vi "calculator.vi"() -> ()   [LabVIEW 2015]
panel:
  out "time to use(s)":dbl
  in  "1":bool
  in  "stop":bool
  in  "CE":bool
  in  "backspace":bool
  in  "1/x":bool
  in  "+/-":bool
  in  "sqrt":bool
  in  ".":bool
  out "message":string
  out "show":string
  in  "C":bool
  out "Current Time":timestamp
  in  "=":bool
  in  "/":bool
  in  "*":bool
  in  "-":bool
  in  "+":bool
  in  "0":bool
  in  "9":bool
  in  "8":bool
  in  "7":bool
  in  "6":bool
  in  "5":bool
  in  "4":bool
  in  "3":bool
  in  "2":bool
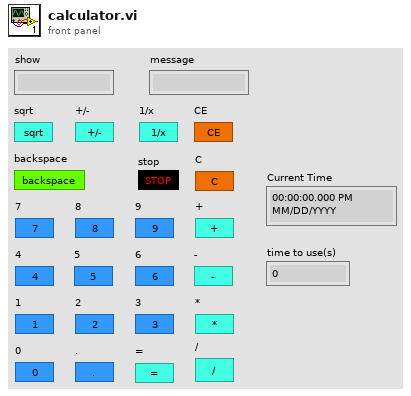
[diagram p1: front panel]
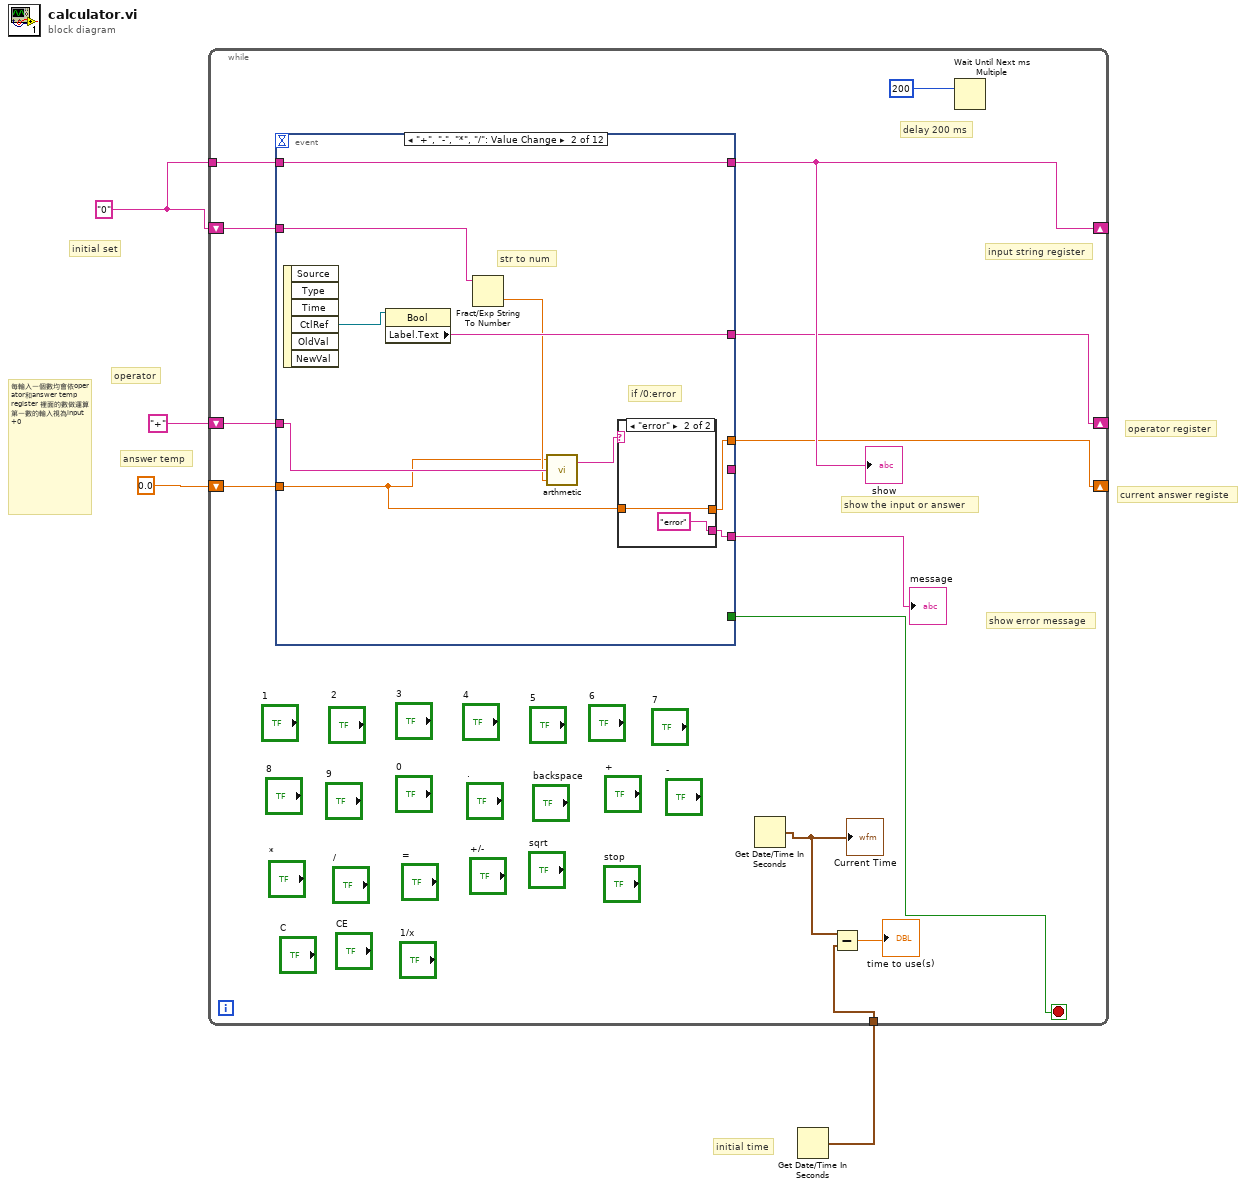
[diagram p0: block diagram]
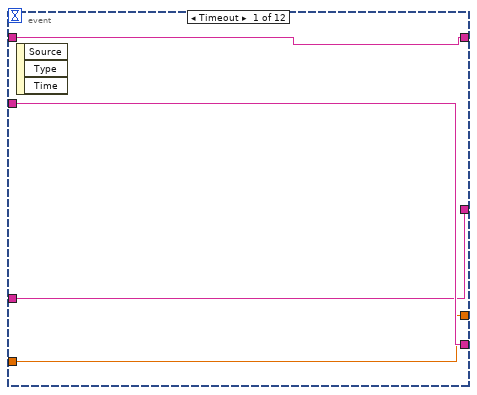
[diagram p2: hidden frame]
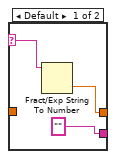
[diagram p3: hidden frame]
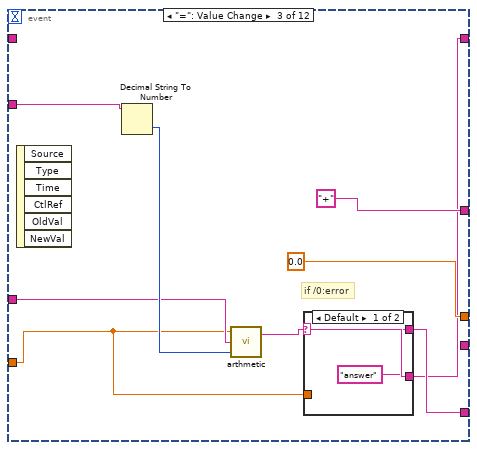
[diagram p4: hidden frame]
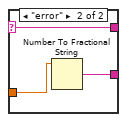
[diagram p5: hidden frame]
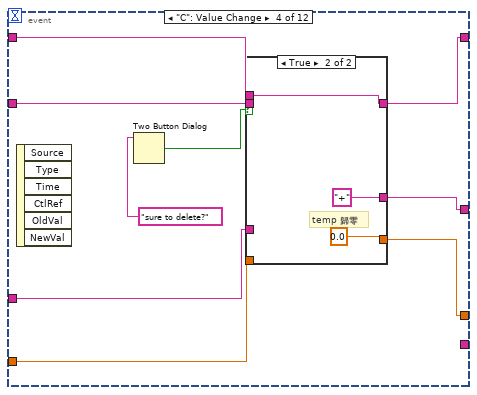
[diagram p6: hidden frame]
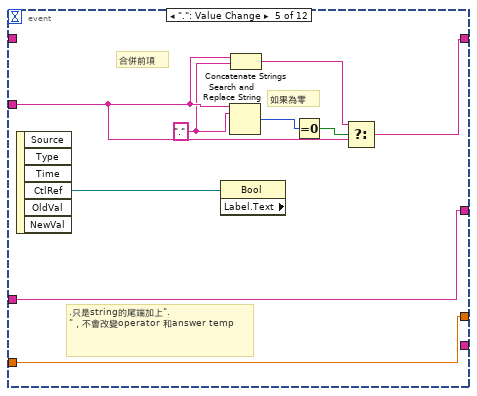
[diagram p8: hidden frame]
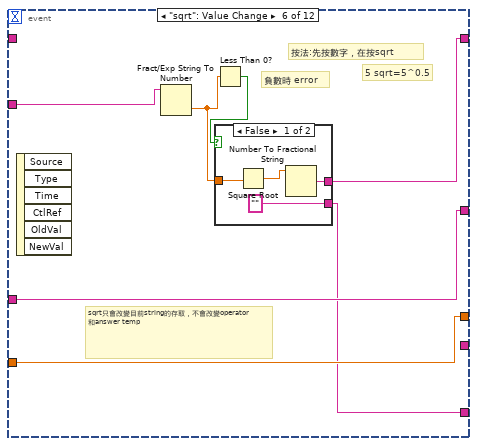
[diagram p9: hidden frame]
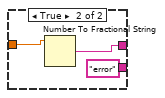
[diagram p10: hidden frame]
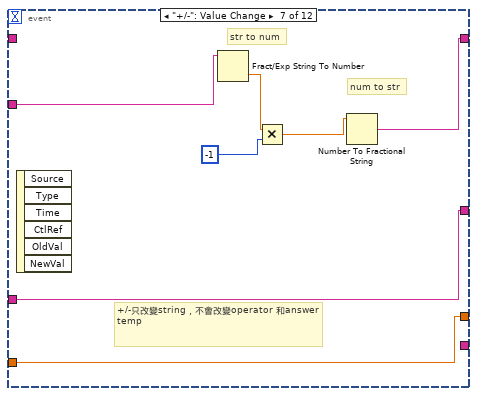
[diagram p11: hidden frame]
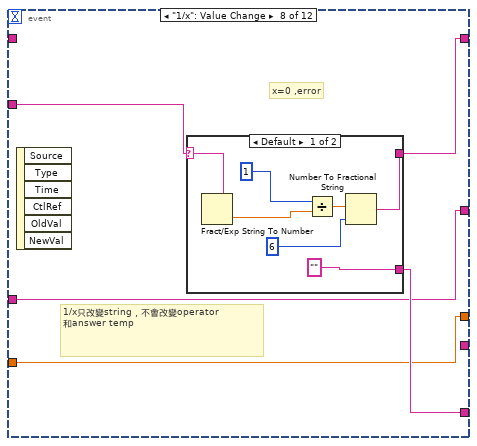
[diagram p12: hidden frame]
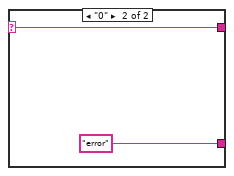
[diagram p13: hidden frame]
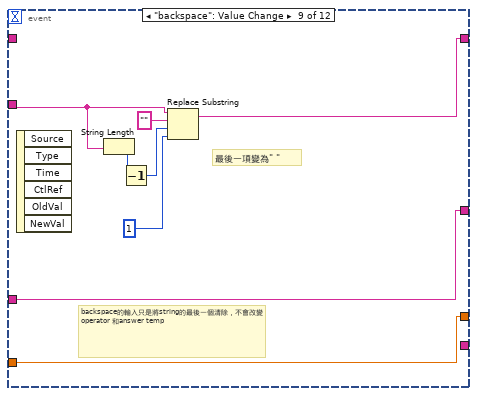
[diagram p14: hidden frame]
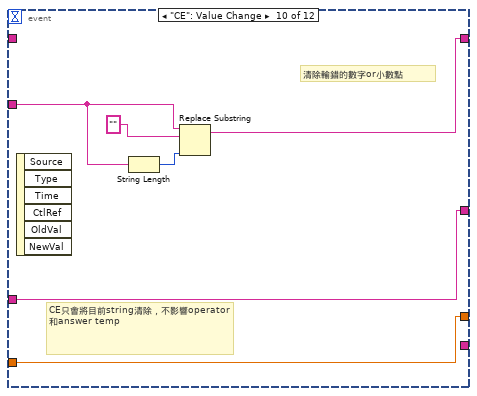
[diagram p15: hidden frame]
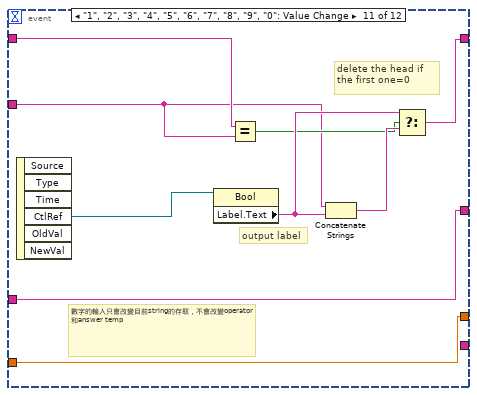
[diagram p16: hidden frame]
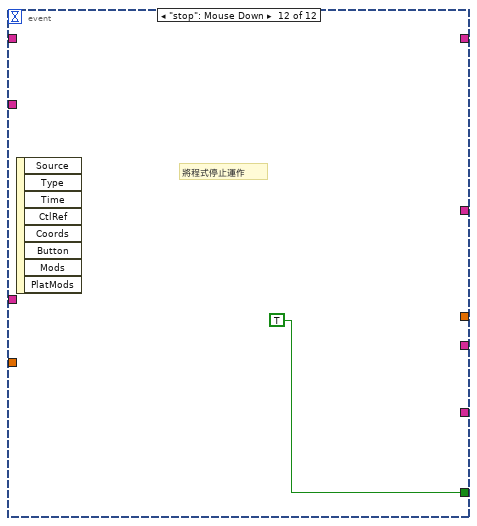
[diagram p17: hidden frame]
diagram:
  w3 = "0"
  # "每輸入一個數均會依operator和answer temp register 裡面的數做運算\n第一數的輸入視為input+0"
  # "current answer registe"
  # "operator register"
  # "answer temp"
  # "operator"
  # "initial time"
  # "initial set"
  n1 = Get Date/Time In Seconds() -> (seconds since 1Jan1904=w4:timestamp)
  n2 = while {
    shift-right: [w11] -> _
    shift-left: w3 -> [w17]
    tunnel: w4 -> [w16]
    tunnel: w3 -> [w12]
    shift-right: [w6] -> _
    shift-left: "+" -> [w10]
    shift-right: [w7] -> _
    shift-left: 0.0 -> [w8]
    stop <- w5 stop-if-true
    # "input string register"
    # "show error message"
    # "show the input or answer"
    # "delay 200 ms"
    n3 = event shown="[1] \"+\", \"-\", \"*\", \"/\": Value Change" {
      selector: _ -> [_ _ _ _ _ _ _ _ _ _ _ _]
      dyn-events: _ -> [_ _ _ _ _ _ _ _ _ _ _ _]
      timeout: _ -> [_ _ _ _ _ _ _ _ _ _ _ _]
      tunnel: w17 -> [w21 w31 w45 w57 w69 w79 w91 w100 w114 w119 w127 _]
      tunnel: w12 -> [w20 w30 _ w55 _ _ _ _ _ _ w128 _]
      tunnel: [w20 w30 w37 w56 w71 w76 w94 w98 w116 w118 w126 _] -> w11
      tunnel: [w21 _ _ _ _ _ _ _ _ _ _ _] -> _
      tunnel: w10 -> [w19 w28 w41 w52 w67 w81 w90 w97 w111 w123 w125 _]
      tunnel: [_ w26 w39 _ _ w75 _ w99 _ _ _ _] -> w9
      tunnel: w8 -> [w18 w22 w38 w51 w66 w80 w89 w96 w110 w122 w124 _]
      tunnel: [w18 w25 0.0 w53 w66 w80 w89 w96 w110 w122 w124 _] -> w7
      tunnel: [w19 w27 "+" w54 w67 w81 w90 w97 w111 w123 w125 _] -> w6
      tunnel: [_ _ _ _ _ _ _ _ _ _ _ TRUE] -> w5
      event Timeout {
        n4 = event-data() -> ()  [unwired: 1 in, 3 out]
      }
      event "+", "-", "*", "/": Value Change {
        # "if /0:error"
        # "str to num"
        n5 = event-data() -> ("CtlRef"=w29:refnum<vi>)  [unwired: 1 in, 5 out]
        n6 = property class="Bool"(reference=w29) -> ("Label.Text"=w27:string)  [unwired: 1 in, 2 out]
        n7 = Fract/Exp String To Number(string=w31) -> (number=w24:dbl)  [unwired: 3 in, 1 out]
        n8 = call "arthmetic.vi"("Numeric 2"=w24, "operator"=w28, "Numeric"=w22) -> ("String 2"=w23:string)  [unwired: 1 in]
        n9 = case shown="\"error\"" w23 {
          selector: w23 -> [w32 _]
          tunnel: ["" "error"] -> w26
          tunnel: [w34 w35] -> w25
          tunnel: w22 -> [_ w35]
          frame Default {
            n10 = Fract/Exp String To Number(string=w32) -> (number=w34:dbl)  [unwired: 3 in, 1 out]
          }
          frame "error" {
          }
        }
      }
      event "=": Value Change {
        # "if /0:error"
        n11 = event-data() -> ()  [unwired: 1 in, 6 out]
        n12 = Decimal String To Number(string=w45) -> (number=w42:i32)  [unwired: 2 in, 1 out]
        n13 = call "arthmetic.vi"("Numeric 2"=w42, "operator"=w41, "Numeric"=w38) -> ("String 2"=w40:string)  [unwired: 1 in]
        n14 = case shown="Default" w40 {
          selector: w40 -> [w47 w50]
          tunnel: ["answer" w50] -> w39
          tunnel: w38 -> [_ w49]
          tunnel: [w47 w48] -> w37
          frame Default {
          }
          frame "error" {
            n15 = Number To Fractional String(number=w49) -> (F-format string=w48:string)  [unwired: 3 in]
          }
        }
      }
      event "C": Value Change {
        n16 = event-data() -> ()  [unwired: 1 in, 6 out]
        n17 = Two Button Dialog(message="sure to delete?") -> (T button?=w58:bool)  [unwired: 2 in]
        n18 = case shown="True" w58 {
          tunnel: w57 -> [w62 _]
          tunnel: [w62 w65] -> w56
          tunnel: w55 -> [_ w65]
          tunnel: [w61 "+"] -> w54
          tunnel: [w60 0.0] -> w53
          tunnel: w52 -> [w61 _]
          tunnel: w51 -> [w60 _]
          frame False {
            # "不清除保留原本資料"
          }
          frame True {
            # "temp 歸零"
          }
        }
      }
      event ".": Value Change {
        w68 = "."
        # ".只是string的尾端加上\".\"，不會改變operator 和answer temp"
        # "如果為零"
        # "合併前項"
        n19 = event-data() -> ("CtlRef"=w74:refnum<vi>)  [unwired: 1 in, 5 out]
        n20 = property class="Bool" props=["Label", "Text"](reference=w74) -> ()  [unwired: 1 in, 3 out]
        n21 = Search and Replace String(input string=w69, search string=w68) -> (number of replacements=w73:i32)  [unwired: 6 in, 3 out]
        n22 = Concatenate Strings(w69, w68) -> (w70:string)
        n23 = Equal To 0?(x=w73) -> (x = 0?=w72:bool)
        n24 = Select(t=w70, s=w72, f=w69) -> (s? t:f=w71:string)
      }
      event "sqrt": Value Change {
        # "sqrt只會改變目前string的存取，不會改變operator 和answer temp"
        # "負數時 error"
        # "按法:先按數字，在按sqrt"
        # "5 sqrt=5^0.5"
        n25 = event-data() -> ()  [unwired: 1 in, 6 out]
        n26 = Fract/Exp String To Number(string=w79) -> (number=w77:dbl)  [unwired: 3 in, 1 out]
        n27 = Less Than 0?(x=w77) -> (x < 0?=w78:bool)
        n28 = case shown="False" w78 {
          tunnel: w77 -> [w85 w88]
          tunnel: [w83 w87] -> w76
          tunnel: ["" "error"] -> w75
          frame False {
            n29 = Square Root(x=w85) -> (sqrt(x)=w84:dbl)
            n30 = Number To Fractional String(number=w84) -> (F-format string=w83:string)  [unwired: 3 in]
          }
          frame True {
            n31 = Number To Fractional String(number=w88) -> (F-format string=w87:string)  [unwired: 3 in]
          }
        }
      }
      event "+/-": Value Change {
        # "+/-只改變string，不會改變operator 和answer temp"
        # "num to str"
        # "str to num"
        n32 = event-data() -> ()  [unwired: 1 in, 6 out]
        n33 = Fract/Exp String To Number(string=w91) -> (number=w93:dbl)  [unwired: 3 in, 1 out]
        n34 = Multiply(x=w93, y=-1) -> (x*y=w92:dbl)
        n35 = Number To Fractional String(number=w92) -> (F-format string=w94:string)  [unwired: 3 in]
      }
      event "1/x": Value Change {
        # "1/x只改變string，不會改變operator 和answer temp"
        # "x=0 ,error"
        n36 = event-data() -> ()  [unwired: 1 in, 6 out]
        n37 = case shown="Default" w100 {
          selector: w100 -> [w107 w108]
          tunnel: ["" "error"] -> w99
          tunnel: [w102 w108] -> w98
          frame Default {
            n38 = Fract/Exp String To Number(string=w107) -> (number=w105:dbl)  [unwired: 3 in, 1 out]
            n39 = Divide(x=1, y=w105) -> (x/y=w103:dbl)
            n40 = Number To Fractional String(number=w103, precision (6)=6) -> (F-format string=w102:string)  [unwired: 2 in]
          }
          frame "0" {
          }
        }
      }
      event "backspace": Value Change {
        # "backspace的輸入只是將string的最後一個清除，不會改變operator 和answer temp"
        # "最後一項變為\" \""
        n41 = event-data() -> ()  [unwired: 1 in, 6 out]
        n42 = String Length(string=w114) -> (length=w113:i32)
        n43 = Decrement(x=w113) -> (x-1=w112:i32)
        n44 = Replace Substring(2:1, 3:w112, 4:"", 5:w114) -> (1:w116:string)  [unwired: 1 out]
      }
      event "CE": Value Change {
        # "CE只會將目前string清除，不影響operator 和answer temp"
        # "清除輸錯的數字or小數點"
        n45 = event-data() -> ()  [unwired: 1 in, 6 out]
        n46 = String Length(string=w119) -> (length=w120:i32)
        n47 = Replace Substring(2:w120, 4:"", 5:w119) -> (1:w118:string)  [unwired: 1 in, 1 out]
      }
      event "1", "2", "3", "4", "5", "6", "7", "8", "9", "0": Value Change {
        # "數字的輸入只會改變目前string的存取，不會改變operator 和answer temp"
        # "output label"
        # "delete the head if the first one=0"
        n48 = event-data() -> ("CtlRef"=w132:refnum<vi>)  [unwired: 1 in, 5 out]
        n49 = property class="Bool"(reference=w132) -> ("Label.Text"=w131:string)  [unwired: 1 in, 2 out]
        n50 = Equal?(x=w128, y=w127) -> (x = y?=w129:bool)
        n51 = Concatenate Strings(w127, w131) -> (w130:string)
        n52 = Select(t=w131, s=w129, f=w130) -> (s? t:f=w126:string)
      }
      event "stop": Mouse Down {
        # "將程式停止運作"
        n53 = event-data() -> ()  [unwired: 1 in, 8 out]
      }
    }
    "show" <- w11
    "message" <- w9
    n54 = Get Date/Time In Seconds() -> (seconds since 1Jan1904=w15:timestamp)
    "Current Time" <- w15
    n55 = Subtract(x=w15, y=w16) -> (x-y=→"time to use(s)":dbl)
    n56 = Wait Until Next ms Multiple(millisecond multiple=200) -> ()  [unwired: 1 out]
  }
